vi "Get Position Count.vi"(8 "error in (no error)":errorcluster, 11 "FW102C in":i32) -> (0 "error out":errorcluster, 2 "Position Count":i32, 3 "FW102C out":i32)   [LabVIEW 2018, in "Thorlabs_FW102C.lvlib"]
doc: "Returns the wheel type"
uses:
  Thorlabs_FW102C.lvlib
  <instrlib>/Thorlabs_FW102C/Library/FilterWheel102_win32.dll
  Library/FilterWheel102_win64.dll
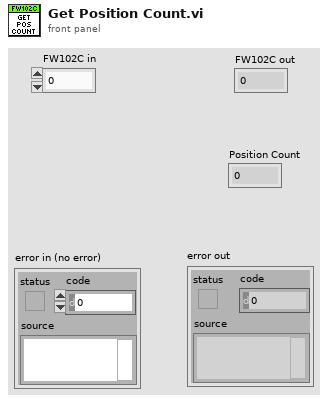
[diagram p1: front panel]
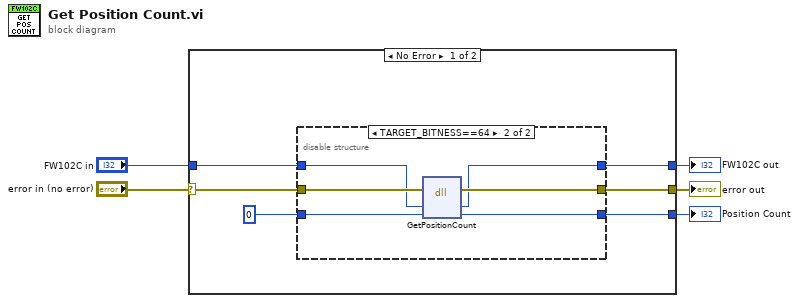
[diagram p0: block diagram]
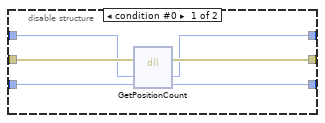
[diagram p2: hidden frame]
diagram:
  n1 = case shown="No Error" "error in (no error)" {
    selector: "error in (no error)" -> [w11 w24]
    tunnel: [w10 w24] -> w5
    tunnel: "FW102C in" -> [w9 w25]
    tunnel: [w8 w25] -> w2
    tunnel: [w7 _] -> w1
    frame No Error {
      n2 = disable-structure shown="TARGET_BITNESS==64" {
        disable-tunnel: w11 -> [w17 w23]
        disable-tunnel: [w16 w22] -> w10
        disable-tunnel: w9 -> [w15 w21]
        disable-tunnel: [w14 w20] -> w8
        disable-tunnel: [w13 w19] -> w7
        disable-tunnel: 0 ("position count") -> [w12 w18]
        frame condition #0 {
          n3 = dll-call lib="E:/Program Files (x86)/National Instruments/LabVIEW 2011/instr.lib/Thorlabs_FW102C/Library/FilterWheel102_win32.dll" fn="GetPositionCount"(error in=w17, "hdl"=w15, "position count"=w12) -> (error out=w16:errorcluster, "hdl"=w14:i32, "position count"=w13:i32)  [unwired: 3 in, 1 out]
        }
        frame condition #1 (active) {
          n4 = dll-call lib="C:/Users/astrolab/Desktop/Labview_code/Thorlabs_FW102C/Library/FilterWheel102_win64.dll" fn="GetPositionCount"(error in=w23, "hdl"=w21, "position count"=w18) -> (error out=w22:errorcluster, "hdl"=w20:i32, "position count"=w19:i32)  [unwired: 3 in, 1 out]
        }
      }
    }
    frame Error {
    }
  }
  "error out" <- w5
  "FW102C out" <- w2
  "Position Count" <- w1
